vi "CANopen Configure Device By SDO.vi"() -> ()   [LabVIEW 2016]
doc: "This example demonstrates how to configure device properties by SDOs, and how to read heartbeat messages and PDO messages received periodically from the device."
uses:
  <vilib>/userdefined/High Color/nirio_resource_hc.ctl
  <vilib>/Platform/TimedLoop/XDataNode/timing_clust.ctl
  <vilib>/Platform/TimedLoop/XDataNode/nitl_modes.ctl
  <vilib>/Platform/TimedLoop/XDataNode/wakeup.ctl
  <vilib>/FPGAPlugInAG/cRIO-9033/niLvFpga_Open_cRIO-9033.vi
  <vilib>/rvi/interface/common/dynamic/niFpgaDynamicAddResources.vi
  <vilib>/CANopenLib/CANOPEN.llb/CANopen Interface Create.vi
  <vilib>/CANopenLib/CANOPEN.llb/CANopen Heartbeat Create.vi
  <vilib>/CANopenLib/CANOPEN.llb/CANopen SDO Create.vi
  <vilib>/CANopenLib/CANOPEN.llb/CANopen SDO Write [U16].vi
  <vilib>/CANopenLib/CANOPEN.llb/CANopen SDO Write [U8].vi
  <vilib>/CANopenLib/CANOPEN.llb/CANopen SDO Close.vi
  <vilib>/CANopenLib/CANOPEN.llb/CANopen TPDO Create.vi
  <vilib>/CANopenLib/CANOPEN.llb/CANopen TPDO Start.vi
  <vilib>/CANopenLib/CANOPEN.llb/CANopen Heartbeat State Read.vi
  <vilib>/CANopenLib/CANOPEN.llb/CANopen TPDO Close.vi
  <vilib>/CANopenLib/CANOPEN.llb/CANopen Heartbeat Close.vi
  <vilib>/CANopenLib/CANOPEN.llb/CANopen Interface Close.vi
  <vilib>/FPGAPlugInAG/Dynamic/niLvFpga_Close_Dynamic.vi
  <vilib>/rvi/interface/nirviOpenFPGA/nirviOpenFPGA.xnode
  FPGA Bitfiles/project_FPGATarget_MainFPGA_S9ZLErdeBuw.lvbitx
  FPGA/MainFPGA.vi
  <vilib>/Platform/TimedLoop/XDataNode/XDataNode.xnode
  <vilib>/rvi/interface/nirviCloseFPGA/nirviCloseFPGA.xnode
  <vilib>/Platform/TimedLoop/XDataNode/XDNodeRunTimeDep.lvlib
panel:
  in  "error in":errorcluster
  out "TPDO data":u8[](array[numeric])
  in  "period (ms)":i64=10
  in  "consumer time (ms)":u16=10
  in  "Stop":bool
  out "state":u16(ring) items=["unknown"=1, "boot-up"=0, "stopped"=4, "operational"=5, "pre-operational"=127, "connection lost"=128]
  out "Is new?":bool
  in  "node-ID":u8=1 min=1 max=127 step=1
  in  "baud rate":u32(ring)=2 items=["1 Mbit/s"=0, "800 kbit/s"=1, "500 kbit/s"=2, "250 kbit/s"=3, "125 kbit/s"=4, "50 kbit/s"=6, "20 kbit/s"=7, "10 kbit/s"=8]
  in  "CANopen interface":u32(ring) items=["CANopen01", "CANopen02", "CANopen03", "CANopen04", "CANopen05", "CANopen06", "CANopen07", "CANopen08", "CANopen09", "CANopen10", "CANopen11", "CANopen12", "CANopen13", "CANopen14", "CANopen15", "CANopen16", "CANopen17", "CANopen18", "CANopen19", "CANopen20", "CANopen21", "CANopen22", "CANopen23", "CANopen24", "CANopen25", "CANopen26", "CANopen27", "CANopen28", "CANopen29", "CANopen30", "CANopen31", "CANopen32"]
  # "Overview: This example demonstrates how to configure device properties by SDOs, and how to read Heartbeat messages \nand PDO messages received periodically from the device.\nRequirements: Connect CANopen module with a slave device. \nInstructions:\n1. Specify the values of CANopen interface, baud rate of the CANopen interface, node-ID of the slave device and \n    consumer time (ms) of Heartbeat object.\n2. Run this VI.\n3. Click STOP to stop the VI."
  # "Configure the device"
  # "Read Heartbeat messages and TPDO messages periodically from the device"
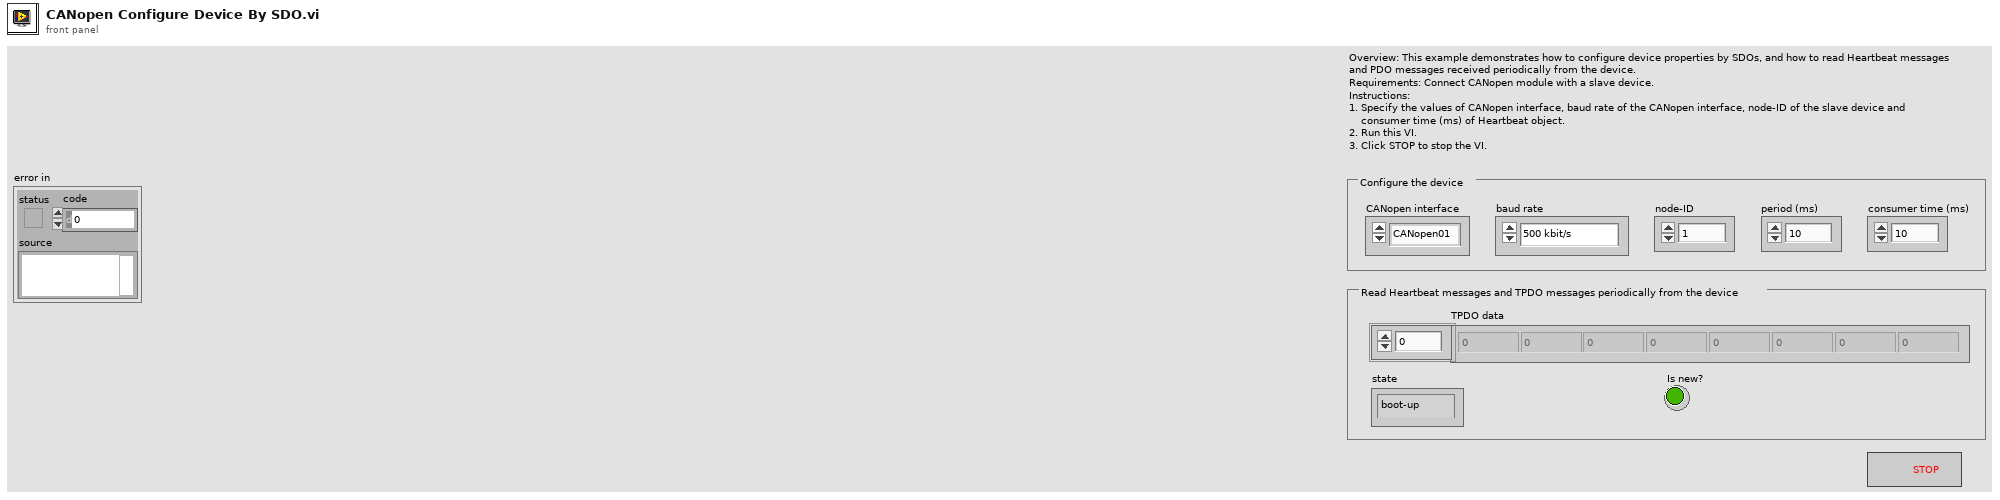
[diagram p1: front panel]
types:
  T1 = typedef "nirio_resource_hc.ctl" = tag
  T2 = typedef "XDNodeRunTimeDep.lvlib/timing_clust.ctl" = cluster{"Expected End [f-1]":u64, "Actual End [f-1]":u64, "Finished Late? [f-1]":bool, "Expected End [i-1]":u64, "Actual End [i-1]":u64, "Finished Late? [i-1]":bool, "Expected Start [i]":u64, "Actual Start [i]":u64, "Expected Start [f]":u64, "Actual Start [f]":u64, "Source Name":string, "Structure Name":string, "Period":i64, "Deadline":i64, "Offset":i64, "Start":i64, "Priority":i32, "Timeout":i32, "Mode":T3, "Wakeup Reason":T4, "Error":errorcluster, "Source Type":string, "Secondary Source Type":string, "Global End Time":u64, "Global Start Time":u64, "Frame Duration":u64, "Iteration Duration":u64, "Assigned CPU":i32, "I/O Scan Engine Mode":u32}
  T3 = typedef "XDNodeRunTimeDep.lvlib/nitl_modes.ctl" = enum32{"No Change", "Process missed periods, maintain original phase", "Discard missed periods, maintain original phase", "Process missed periods, ignore original phase", "Discard missed periods, ignore original phase"}
  T4 = typedef "XDNodeRunTimeDep.lvlib/wakeup.ctl" = enum32{"Normal", "Aborted", "Asynchronous wakeup", "Timing source error", "Timed loop error", "Timeout"}
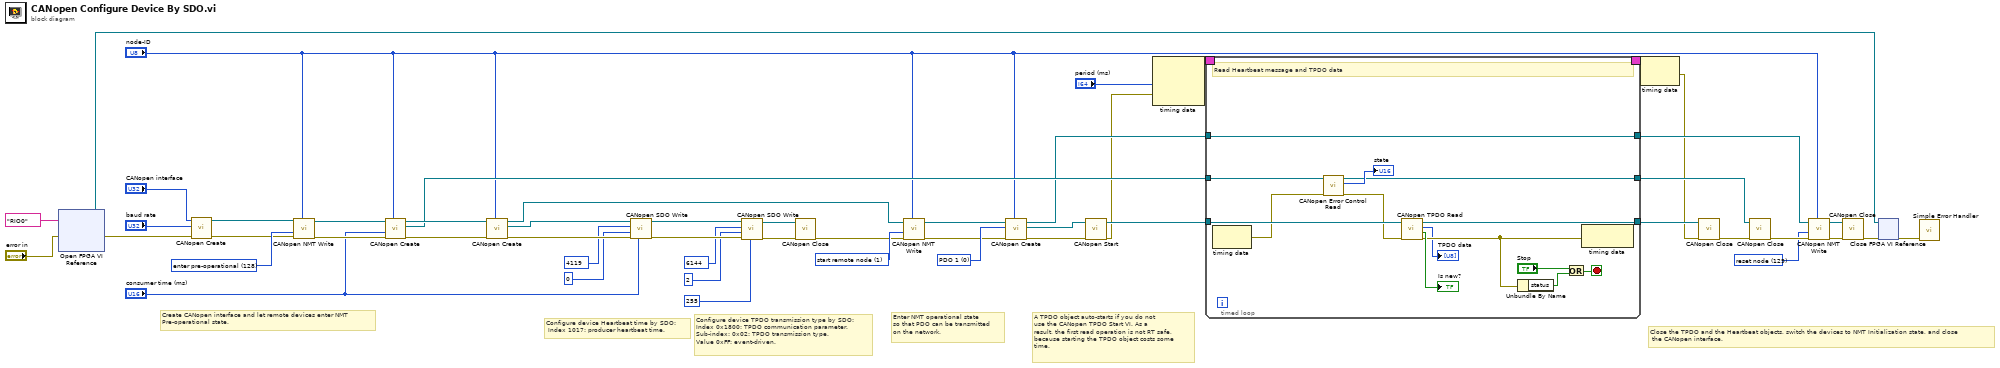
[diagram p0: block diagram]
diagram:
  w12 = u16 129 items=["start remote node"=1, "stop remote node"=2, "enter pre-operational"=128, "reset node"=129, "reset communication"=130] ("command")
  w26 = u16 1 items=["start remote node"=1, "stop remote node"=2, "enter pre-operational"=128, "reset node"=129, "reset communication"=130] ("command")
  w35 = u8 0 items=["PDO 1", "PDO 2", "PDO 3", "PDO 4"] ("PDO Channel")
  w48 = u16 128 items=["start remote node"=1, "stop remote node"=2, "enter pre-operational"=128, "reset node"=129, "reset communication"=130] ("command")
  # "Close the TPDO and the Heartbeat objects, switch the devices to NMT Initialization state, and close\n the CANopen interface."
  # "Create CANopen interface and let remote devices enter NMT\nPre-operational state."
  # "Enter NMT operational state\nso that PDO can be transmitted \non the network."
  # "A TPDO object auto-starts if you do not \nuse the CANopen TPDO Start VI. As a \nresult, the first read operation is not RT safe, \nbecause starting the TPDO object costs some \ntime."
  # "Configure device TPDO transmission type by SDO:\nIndex 0x1800: TPDO communication parameter.\nSub-index: 0x02: TPDO transmission type.\nValue 0xFF: event-driven."
  # "Configure device Heartbeat time by SDO:\n Index 1017: producer heartbeat time."
  n1 = xnode ("Open FPGA VI Reference")("error in"="error in", "resource name"=T1 "RIO0") -> ("FPGA VI Reference Out"=w1:refnum<k20>, "error out"=w4:errorcluster)
  n2 = call-poly <vilib>:"CANopen Create.vi"("error in (no error)"=w4, "baud rate"="baud rate", "interface name"="CANopen interface") -> ("error out"=w47:errorcluster, "interface object out"=w46:refnum<k20>)  [unwired: 7 in]
  n3 = call <vilib>:"CANopen NMT Write.vi"("node-ID (0)"="node-ID", "error in (no error)"=w47, "command"=w48, "interface object in"=w46) -> ("error out"=w44:errorcluster, "interface object out"=w42:refnum<k20>)  [unwired: 6 in]
  n4 = call-poly <vilib>:"CANopen Create.vi"("node-ID"="node-ID", "error in (no error)"=w44, "consumer time [ms]"="consumer time (ms)", "interface object in"=w42) -> ("error out"=w43:errorcluster, "heartbeat object out"=w36:refnum<k20>, "interface object out"=w41:refnum<k20>)  [unwired: 5 in]
  n5 = call-poly <vilib>:"CANopen Create.vi"("node-ID"="node-ID", "error in (no error)"=w43, "interface object in"=w41) -> ("error out"=w39:errorcluster, "SDO object out"=w40:refnum<k20>, "interface object out"=w25:refnum<k20>)  [unwired: 6 in]
  n6 = call-poly <vilib>:"CANopen SDO Write.vi"("U16 data"="consumer time (ms)", "error in (no error)"=w39, "object sub-index (0)"=u8 0, "object index"=u16 4119, "SDO object in"=w40) -> ("error out"=w32:errorcluster, "SDO object out"=w31:refnum<k20>)  [unwired: 4 in, 1 out]
  n7 = call-poly <vilib>:"CANopen SDO Write.vi"("U8 data"=u8 255 ("U32 data"), "error in (no error)"=w32, "object sub-index (0)"=u8 2, "object index"=u16 6144, "SDO object in"=w31) -> ("error out"=w22:errorcluster, "SDO object out"=w23:refnum<k20>)  [unwired: 4 in, 1 out]
  n8 = call-poly <vilib>:"CANopen Close.vi"("error in (no error)"=w22, "SDO object in"=w23) -> ("error out"=w21:errorcluster)  [unwired: 9 in]
  n9 = call <vilib>:"CANopen NMT Write.vi"("node-ID (0)"="node-ID", "error in (no error)"=w21, "command"=w26, "interface object in"=w25) -> ("error out"=w27:errorcluster, "interface object out"=w24:refnum<k20>)  [unwired: 6 in]
  n10 = call-poly <vilib>:"CANopen Create.vi"("node-ID"="node-ID", "error in (no error)"=w27, "PDO channel"=w35, "interface object in"=w24) -> ("error out"=w18:errorcluster, "TPDO object out"=w20:refnum<k20>, "interface object out"=w14:refnum<k20>)  [unwired: 5 in]
  n11 = call-poly <vilib>:"CANopen Start.vi"("error in (no error)"=w18, "TPDO object in"=w20) -> ("error out"=w10:errorcluster, "TPDO object out"=w19:refnum<k20>)  [unwired: 8 in]
  n12 = node-c288("period (ms)", w10) -> (w52:T2)  [unwired: 1 in]
  n13 = timed-loop {
    tunnel: [w66] -> w45
    tunnel: w19 -> [w65]
    timing: w52 -> [_]
    timing-out: [_] -> w51
    tunnel: w36 -> [w62]
    tunnel: [w60] -> w33
    tunnel: w14 -> [w56]
    tunnel: [w56] -> w13
    stop <- w59 stop-if-true
    # "Read Heartbeat message and TPDO data"
    n14 = node-c288() -> (w55:errorcluster)  [unwired: 1 in]
    n15 = call-poly <vilib>:"CANopen Error Control Read.vi"("error in (no error)"=w55, "heartbeat object in"=w62) -> ("error out"=w63:errorcluster, "state"=→"state":u16, "heartbeat object out"=w60:refnum<k20>)  [unwired: 6 in, 1 out]
    n16 = call <vilib>:"CANopen TPDO Read.vi"("error in (no error)"=w63, "TPDO object in"=w65) -> ("error out"=w54:errorcluster, "new data?"=→"Is new?":bool, "data"=→"TPDO data":u8[], "TPDO object out"=w66:refnum<k20>)  [unwired: 5 in, 1 out]
    n17 = Unbundle By Name(w54) -> ("status"=w57:bool)
    n18 = Or(x="Stop", y=w57) -> (x .or. y?=w59:bool)
    n19 = node-c288(w54) -> ()  [unwired: 1 out]
  }
  n20 = node-c288(w51) -> (w9:errorcluster)
  n21 = call-poly <vilib>:"CANopen Close.vi"("error in (no error)"=w9, "TPDO object in"=w45) -> ("error out"=w34:errorcluster)  [unwired: 9 in]
  n22 = call-poly <vilib>:"CANopen Close.vi"("error in (no error)"=w34, "heartbeat object in"=w33) -> ("error out"=w17:errorcluster)  [unwired: 9 in]
  n23 = call <vilib>:"CANopen NMT Write.vi"("node-ID (0)"="node-ID", "error in (no error)"=w17, "command"=w12, "interface object in"=w13) -> ("error out"=w16:errorcluster, "interface object out"=w15:refnum<k20>)  [unwired: 6 in]
  n24 = call-poly <vilib>:"CANopen Close.vi"("error in (no error)"=w16, "interface object in"=w15) -> ("error out"=w3:errorcluster)  [unwired: 9 in]
  n25 = xnode "Close FPGA VI Reference"("FPGA VI Reference In"=w1, "error in"=w3) -> ("error out"=w2:errorcluster)
  n26 = call <vilib>:"Simple Error Handler.vi"("error in (no error)"=w2) -> ()  [unwired: 4 in, 5 out]
